vi "SR830Monitor_old.vi"() -> ()   [LabVIEW 2016]
doc: "This VI is an example of storing and recovering data from the SR830 data buffers .\nDATA STORAGE RATE specifes the rate at which data is added to the data buffers .\nSCAN LENGTH specifies the approximate length of the data acquisition scan is seconds .\nPLOT GRAPH, PLOT CH 1 DATA and PLOT CH 2 DATA specify if the respective graphs will be displayed .\nAfter data storage is completed , the channel 1 and channel 2 points are downloaded from the instrument to the CH 1 POINTS and CH 2 POINTS arrays respectively . \nSince data recovered (using the SR830 receive message.vi) is in the string format , this VI requires a considerable amount of time to format the data into an array of floating point numbers . A quicker way would be to store the string in a file and use a CIN to speed up the process ."
uses:
  Global/Global Variables/Data_Display_global.vi
  Instrument_Setup.vi
panel:
  out "AutoSet3":bool=TRUE
  out "AutoSet2":bool=TRUE
  out "AutoSet1":bool=TRUE
  in  "Stopp":bool
  out "error out":T1
  in  "error in":T1
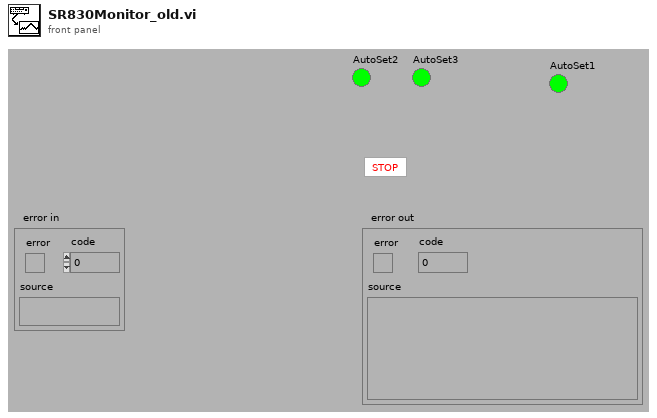
[diagram p1: front panel]
types:
  T1 = cluster{"error":bool, "code":i8, "source":string}
  T2 = cluster{"Lockin1":dbl[], "Lockin3":dbl[], "Lockin2":dbl[]}
  T3 = cluster{"error":bool, "code":i32, "source":string}
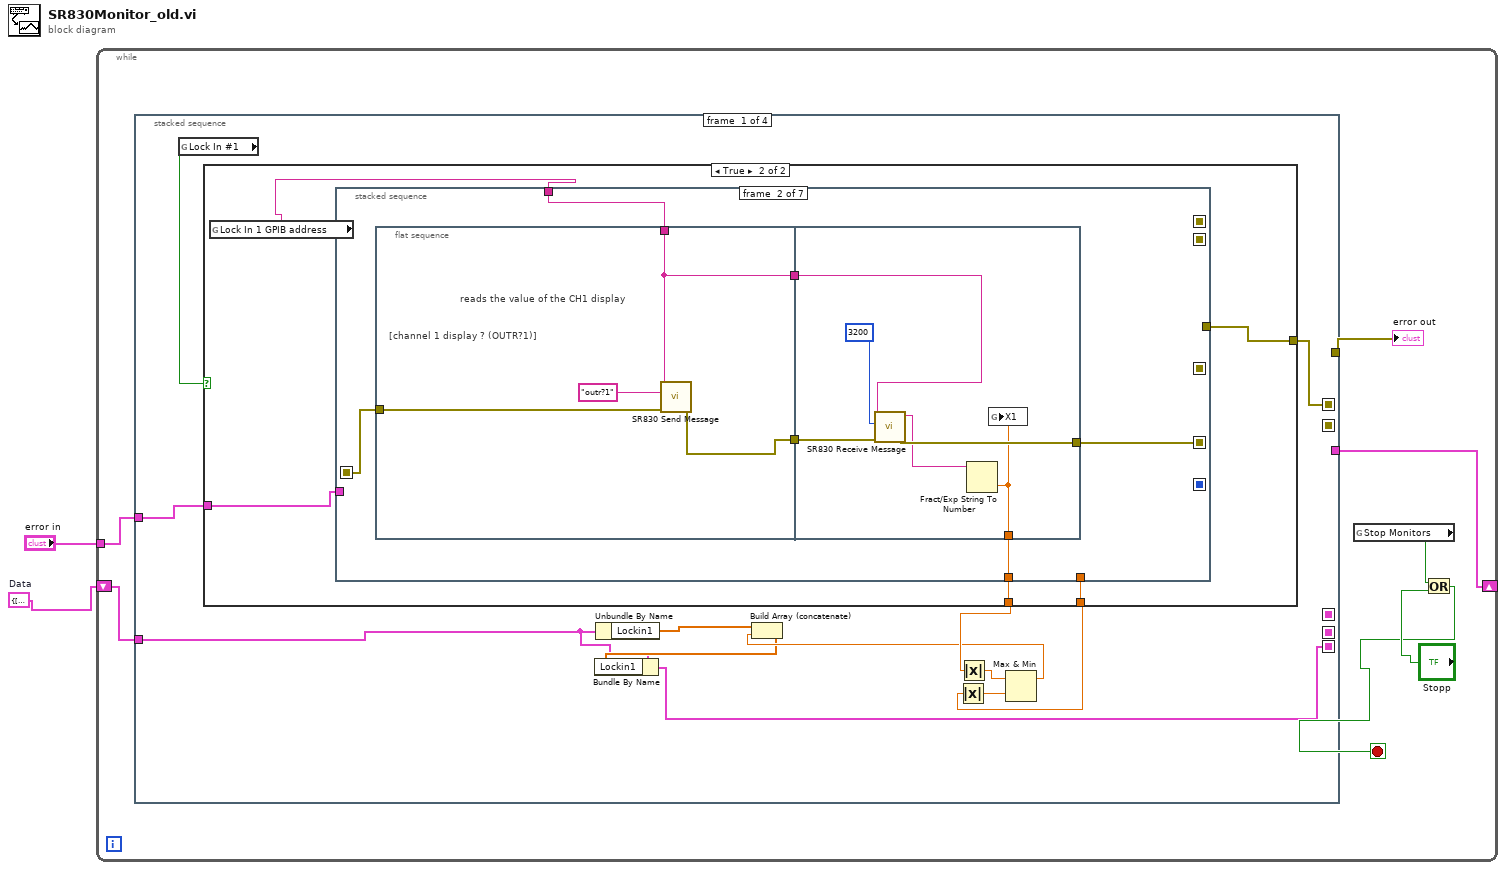
[diagram p0: block diagram]
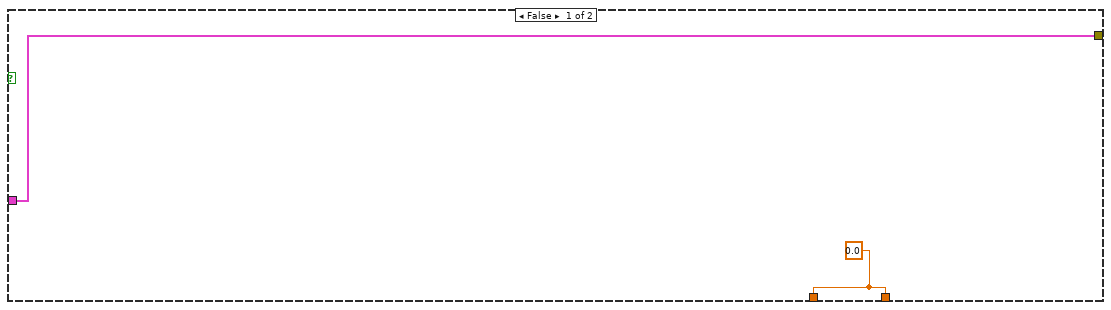
[diagram p2: hidden frame]
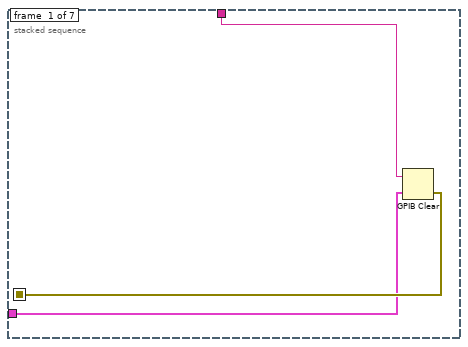
[diagram p3: hidden frame]
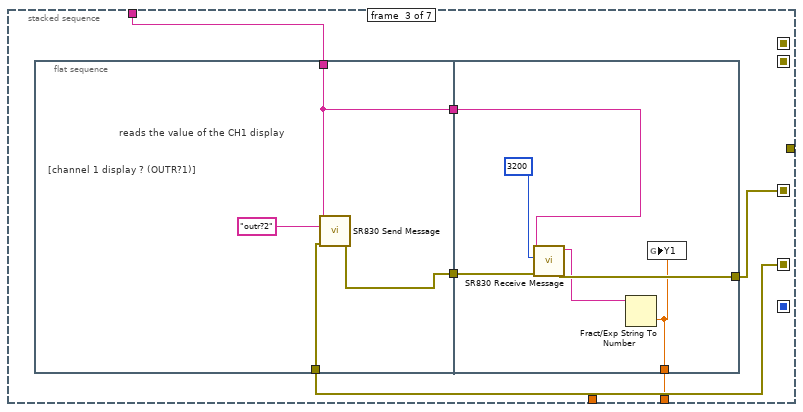
[diagram p4: hidden frame]
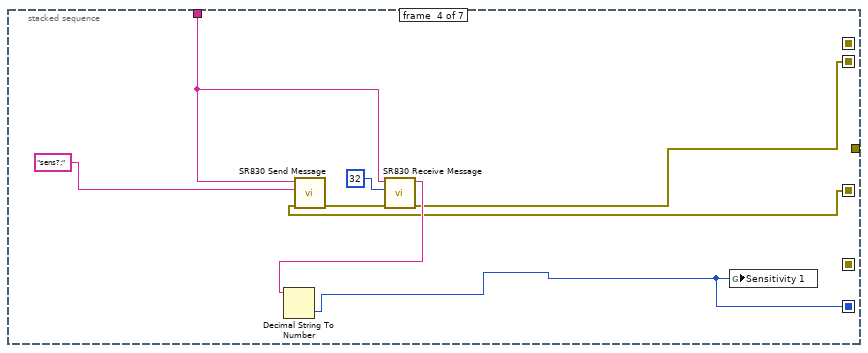
[diagram p5: hidden frame]
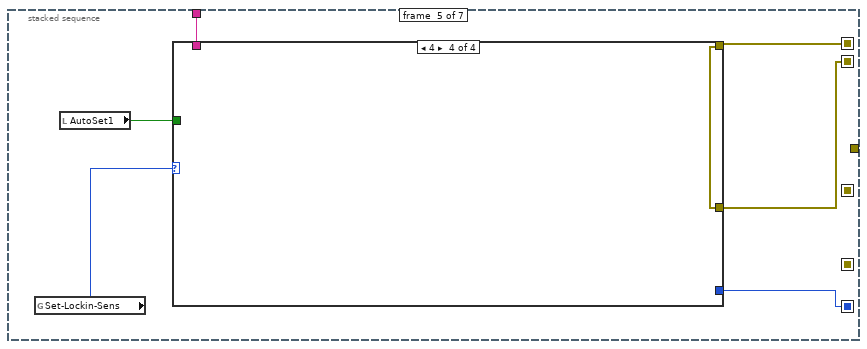
[diagram p6: hidden frame]
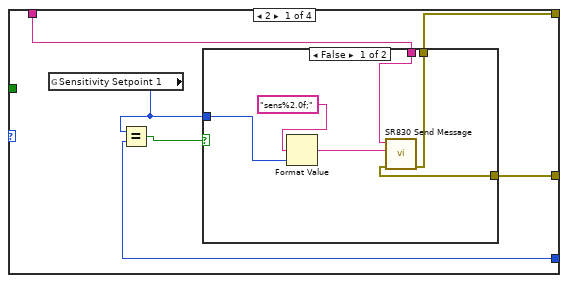
[diagram p7: hidden frame]
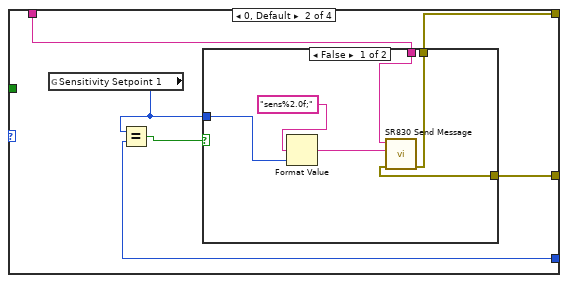
[diagram p9: hidden frame]
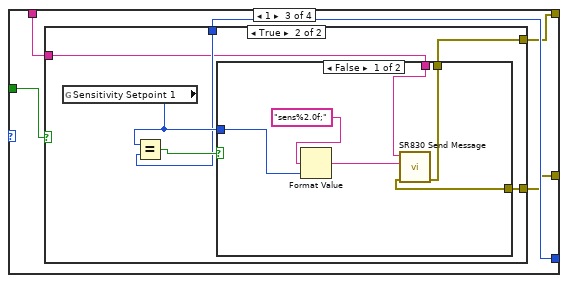
[diagram p11: hidden frame]
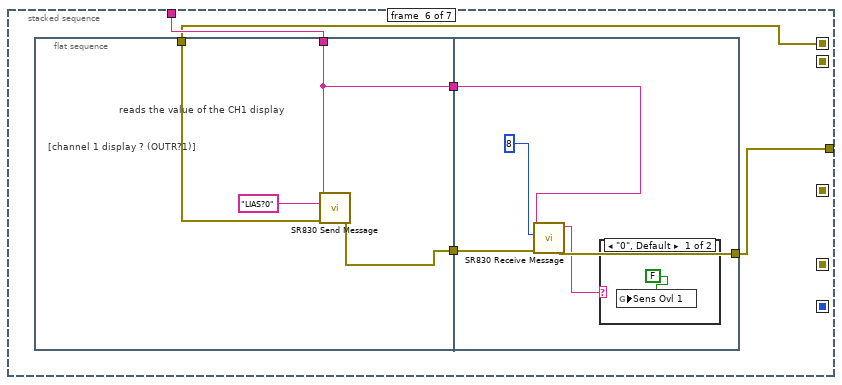
[diagram p14: hidden frame]
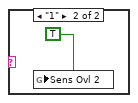
[diagram p15: hidden frame]
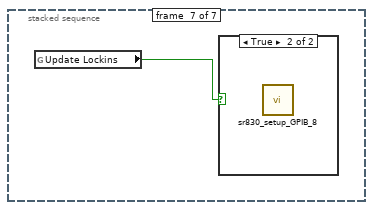
[diagram p16: hidden frame]
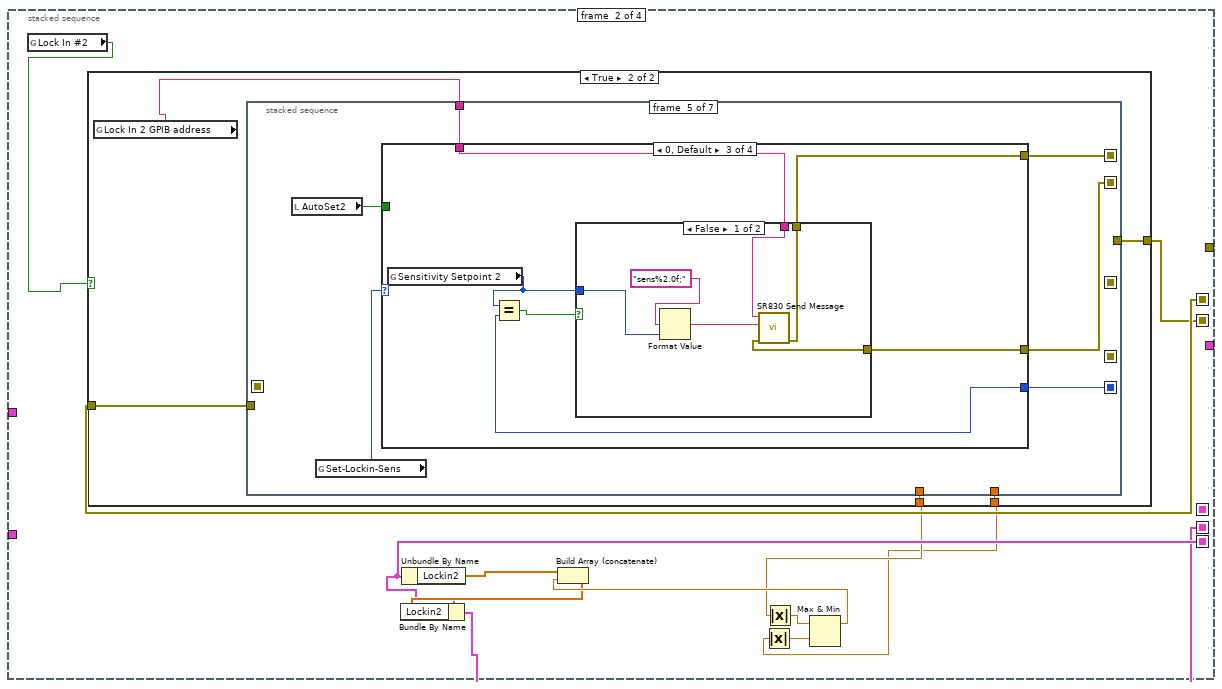
[diagram p18: hidden frame]
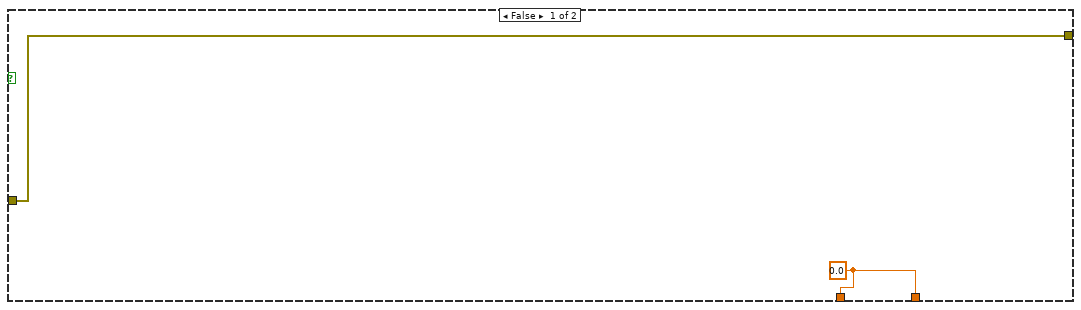
[diagram p19: hidden frame]
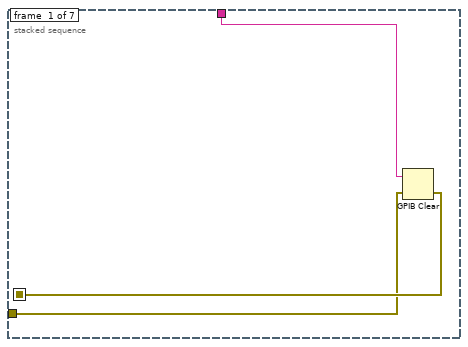
[diagram p20: hidden frame]
diagram:
  w1 = T2 {"Lockin1"=[], "Lockin3"=[], "Lockin2"=[]}  # Data
  n1 = while {
    tunnel: "error in" -> [w9]
    shift-right: [w3] -> _
    shift-left: w1 -> [w4]
    stop <- w5 stop-if-true
    n2 = stacked-sequence {
      seq-local: [w19 _ _ _] -> [_ w152 w284 _]
      seq-local: [_ w150 _ _] -> [_ _ _ _]
      seq-local: [w10 _ _ _] -> [_ w144 _ _]
      seq-local: [_ w141 _ _] -> [_ _ w276 _]
      seq-local: [_ _ w275 _] -> [_ _ _ w391]
      tunnel: w9 -> [w20 _ _ _]
      tunnel: [_ _ w283 _] -> w8
      tunnel: w4 -> [w11 _ _ _]
      tunnel: [_ _ _ w390] -> w3
      frame #0 {
        n3 = global read "Instrument_Setup.vi" "Lock In #1"() -> (w21:bool)
        n4 = case shown="True" w21 {
          tunnel: w20 -> [w23 w28]
          tunnel: [w23 w26] -> w19
          tunnel: [w22 w25] -> w15
          tunnel: [w22 w24] -> w14
          frame False {
            w22 = 0.0
          }
          frame True {
            n5 = global read "Instrument_Setup.vi" "Lock In 1 GPIB address"() -> (w27:string)
            n6 = stacked-sequence {
              seq-local: [_ w34 _ _ _ _ _] -> [_ _ w51 _ _ _ _]
              seq-local: [_ _ w49 _ _ _ _] -> [_ _ _ w66 _ _ _]
              seq-local: [w30 _ _ _ _ _ _] -> [_ w33 _ _ _ _ _]
              seq-local: [_ _ _ w65 _ _ _] -> [_ _ _ _ w77 _ _]
              seq-local: [_ _ _ w64 _ _ _] -> [_ _ _ _ w76 _ _]
              seq-local: [_ _ _ _ w74 _ _] -> [_ _ _ _ _ w124 _]
              tunnel: w27 -> [w31 w37 w50 w68 w75 w126 _]
              tunnel: w28 -> [w29 _ _ _ _ _ _]
              tunnel: [_ _ _ _ _ w125 _] -> w26
              tunnel: [_ w32 _ _ _ _ _] -> w25
              tunnel: [_ _ w48 _ _ _ _] -> w24
              frame #0 {
                n7 = GPIB Clear(2:w29, 3:w31) -> (0:w30:errorcluster)  [unwired: 1 out]
              }
              frame #1 {
                n8 = flat-sequence {
                  tunnel: w37 -> [w40]
                  tunnel: [w40] -> w36
                  tunnel: [w39] -> w35
                  tunnel: w33 -> [w38]
                  tunnel: w36 -> [w46]
                  tunnel: w35 -> [w45]
                  tunnel: [w44] -> w34
                  tunnel: [w42] -> w32
                  frame #0 {
                    # "[channel 1 display ? (OUTR?1)]"
                    # "reads the value of the CH1 display"
                    n9 = call "SR830 Send Message.vi"("address string"=w40, "write buffer"="outr?1", "error in"=w38) -> ("error out"=w39:T3)  [unwired: 4 in, 2 out]
                  }
                  frame #1 {
                    n10 = call "SR830 Receive Message.vi"("address string"=w46, "byte count"=3200, "error in"=w45) -> ("read buffer"=w43:string, "error out"=w44:T3)  [unwired: 4 in, 1 out]
                    n11 = Fract/Exp String To Number(string=w43) -> (number=w42:dbl)  [unwired: 3 in, 1 out]
                    n12 = global write "Data_Display_global.vi" "X1"(w42) -> ()
                  }
                }
              }
              frame #2 {
                n13 = flat-sequence {
                  tunnel: w50 -> [w56]
                  tunnel: [w56] -> w53
                  tunnel: [w55] -> w52
                  tunnel: w51 -> [w54]
                  tunnel: w53 -> [w62]
                  tunnel: w52 -> [w61]
                  tunnel: [w60] -> w49
                  tunnel: [w58] -> w48
                  frame #0 {
                    # "[channel 1 display ? (OUTR?1)]"
                    # "reads the value of the CH1 display"
                    n14 = call "SR830 Send Message.vi"("address string"=w56, "write buffer"="outr?2", "error in"=w54) -> ("error out"=w55:T3)  [unwired: 4 in, 2 out]
                  }
                  frame #1 {
                    n15 = call "SR830 Receive Message.vi"("address string"=w62, "byte count"=3200, "error in"=w61) -> ("read buffer"=w59:string, "error out"=w60:T3)  [unwired: 4 in, 1 out]
                    n16 = Fract/Exp String To Number(string=w59) -> (number=w58:dbl)  [unwired: 3 in, 1 out]
                    n17 = global write "Data_Display_global.vi" "Y1"(w58) -> ()
                  }
                }
              }
              frame #3 {
                n18 = call "SR830 Send Message.vi"("address string"=w68, "write buffer"="sens?;", "error in"=w66) -> ("error out"=w70:T3)  [unwired: 4 in, 2 out]
                n19 = call "SR830 Receive Message.vi"("address string"=w68, "byte count"=32, "error in"=w70) -> ("read buffer"=w67:string, "error out"=w65:T3)  [unwired: 4 in, 1 out]
                n20 = Decimal String To Number(string=w67) -> (number=w64:i32)  [unwired: 2 in, 1 out]
                n21 = global write "Data_Display_global.vi" "Sensitivity 1"(w64) -> ()
              }
              frame #4 {
                n22 = global read "Instrument_Setup.vi" "Set-Lockin-Sens"() -> (w73:u16)
                n23 = local read "AutoSet1"() -> (w72:bool)
                n24 = case shown="4" w73 {
                  tunnel: w77 -> [w81 w94 w104 w123]
                  tunnel: w76 -> [w80 w93 w107 _]
                  tunnel: w75 -> [w79 w92 w106 _]
                  tunnel: [w78 w91 w105 w123] -> w74
                  tunnel: w72 -> [_ _ w108 _]
                  frame 2 {
                    n25 = global read "Data_Display_global.vi" "Sensitivity Setpoint 1"() -> (w82:i32)
                    n26 = Equal?(x=w82, y=w80) -> (x = y?=w83:bool)
                    n27 = case shown="False" w83 {
                      tunnel: w79 -> [w89 _]
                      tunnel: w82 -> [w88 _]
                      tunnel: w81 -> [w87 w90]
                      tunnel: [w86 w90] -> w78
                      frame False {
                        n28 = Format Value(format string="sens%2.0f;", value (0)=w88) -> (output string=w85:string)  [unwired: 1 in]
                        n29 = call "SR830 Send Message.vi"("address string"=w89, "write buffer"=w85, "error in"=w87) -> ("error out"=w86:T3)  [unwired: 4 in, 2 out]
                      }
                      frame True {
                      }
                    }
                  }
                  frame 0, Default {
                    n30 = global read "Data_Display_global.vi" "Sensitivity Setpoint 1"() -> (w95:i32)
                    n31 = Equal?(x=w95, y=w93) -> (x = y?=w96:bool)
                    n32 = case shown="False" w96 {
                      tunnel: w92 -> [w102 _]
                      tunnel: w95 -> [w101 _]
                      tunnel: w94 -> [w100 w103]
                      tunnel: [w99 w103] -> w91
                      frame False {
                        n33 = Format Value(format string="sens%2.0f;", value (0)=w101) -> (output string=w98:string)  [unwired: 1 in]
                        n34 = call "SR830 Send Message.vi"("address string"=w102, "write buffer"=w98, "error in"=w100) -> ("error out"=w99:T3)  [unwired: 4 in, 2 out]
                      }
                      frame True {
                      }
                    }
                  }
                  frame 1 {
                    n35 = case shown="True" w108 {
                      tunnel: w107 -> [_ w113]
                      tunnel: w106 -> [_ w112]
                      tunnel: [w109 w111] -> w105
                      tunnel: w104 -> [w109 w110]
                      frame False {
                      }
                      frame True {
                        n36 = global read "Data_Display_global.vi" "Sensitivity Setpoint 1"() -> (w114:i32)
                        n37 = Equal?(x=w114, y=w113) -> (x = y?=w115:bool)
                        n38 = case shown="False" w115 {
                          tunnel: w112 -> [w121 _]
                          tunnel: w114 -> [w120 _]
                          tunnel: w110 -> [w116 w122]
                          tunnel: [w119 w122] -> w111
                          frame False {
                            n39 = Format Value(format string="sens%2.0f;", value (0)=w120) -> (output string=w118:string)  [unwired: 1 in]
                            n40 = call "SR830 Send Message.vi"("address string"=w121, "write buffer"=w118, "error in"=w116) -> ("error out"=w119:T3)  [unwired: 4 in, 2 out]
                          }
                          frame True {
                          }
                        }
                      }
                    }
                  }
                  frame 4 {
                  }
                }
              }
              frame #5 {
                n41 = flat-sequence {
                  tunnel: w126 -> [w131]
                  tunnel: [w131] -> w128
                  tunnel: [w130] -> w127
                  tunnel: w124 -> [w129]
                  tunnel: w128 -> [w136]
                  tunnel: w127 -> [w135]
                  tunnel: [w134] -> w125
                  frame #0 {
                    # "[channel 1 display ? (OUTR?1)]"
                    # "reads the value of the CH1 display"
                    n42 = call "SR830 Send Message.vi"("address string"=w131, "write buffer"="LIAS?0", "error in"=w129) -> ("error out"=w130:T3)  [unwired: 4 in, 2 out]
                  }
                  frame #1 {
                    n43 = call "SR830 Receive Message.vi"("address string"=w136, "byte count"=8, "error in"=w135) -> ("read buffer"=w133:string, "error out"=w134:T3)  [unwired: 4 in, 1 out]
                    n44 = case shown="\"0\", Default" w133 {
                      frame "0", Default {
                        n45 = global write "Data_Display_global.vi" "Sens Ovl 1"(FALSE) -> ()
                      }
                      frame "1" {
                        n46 = global write "Data_Display_global.vi" "Sens Ovl 2"(TRUE) -> ()
                      }
                    }
                  }
                }
              }
              frame #6 {
                n47 = global read "Instrument_Setup.vi" "Update Lockins"() -> (w140:bool)
                n48 = case shown="True" w140 {
                  frame False {
                  }
                  frame True {
                    n49 = call "sr830_setup_GPIB_8.vi"() -> ()  [unwired: 3 in]
                  }
                }
              }
            }
          }
        }
        n50 = Unbundle By Name(w11) -> ("Lockin1"=w18:dbl[])
        n51 = Absolute Value(x=w14) -> (abs(x)=w16:dbl)
        n52 = Absolute Value(x=w15) -> (abs(x)=w17:dbl)
        n53 = Max & Min(x=w17, y=w16) -> (max(x,y)=w13:dbl)  [unwired: 1 out]
        n54 = Build Array (concatenate)(w18, w13) -> (w12:dbl[])
        n55 = Bundle By Name(cluster=w11, "Lockin1"=w12) -> (w10:T2)
      }
      frame #1 {
        n56 = global read "Instrument_Setup.vi" "Lock In #2"() -> (w151:bool)
        n57 = case shown="True" w151 {
          tunnel: w152 -> [w154 w158]
          tunnel: [w154 w157] -> w150
          tunnel: [w153 w156] -> w143
          tunnel: [w153 w155] -> w142
          frame False {
            w153 = 0.0
          }
          frame True {
            n58 = global read "Instrument_Setup.vi" "Lock In 2 GPIB address"() -> (w159:string)
            n59 = stacked-sequence {
              seq-local: [_ w165 _ _ _ _ _] -> [_ _ w182 _ _ _ _]
              seq-local: [_ _ w180 _ _ _ _] -> [_ _ _ w197 _ _ _]
              seq-local: [w161 _ _ _ _ _ _] -> [_ w164 _ _ _ _ _]
              seq-local: [_ _ _ w196 _ _ _] -> [_ _ _ _ w206 _ _]
              seq-local: [_ _ _ w195 _ _ _] -> [_ _ _ _ w207 _ _]
              seq-local: [_ _ _ _ w205 _ _] -> [_ _ _ _ _ w255 _]
              tunnel: w159 -> [w162 w168 w181 w199 w208 w257 _]
              tunnel: w158 -> [w160 _ _ _ _ _ _]
              tunnel: [_ _ _ _ _ w256 _] -> w157
              tunnel: [_ w163 _ _ _ _ _] -> w156
              tunnel: [_ _ w179 _ _ _ _] -> w155
              frame #0 {
                n60 = GPIB Clear(2:w160, 3:w162) -> (0:w161:errorcluster)  [unwired: 1 out]
              }
              frame #1 {
                n61 = flat-sequence {
                  tunnel: w168 -> [w171]
                  tunnel: [w171] -> w167
                  tunnel: [w170] -> w166
                  tunnel: w164 -> [w169]
                  tunnel: w167 -> [w177]
                  tunnel: w166 -> [w176]
                  tunnel: [w175] -> w165
                  tunnel: [w173] -> w163
                  frame #0 {
                    # "[channel 1 display ? (OUTR?1)]"
                    # "reads the value of the CH1 display"
                    n62 = call "SR830 Send Message.vi"("address string"=w171, "write buffer"="outr?1", "error in"=w169) -> ("error out"=w170:T3)  [unwired: 4 in, 2 out]
                  }
                  frame #1 {
                    n63 = call "SR830 Receive Message.vi"("address string"=w177, "byte count"=3200, "error in"=w176) -> ("read buffer"=w174:string, "error out"=w175:T3)  [unwired: 4 in, 1 out]
                    n64 = Fract/Exp String To Number(string=w174) -> (number=w173:dbl)  [unwired: 3 in, 1 out]
                    n65 = global write "Data_Display_global.vi" "X2"(w173) -> ()
                  }
                }
              }
              frame #2 {
                n66 = flat-sequence {
                  tunnel: w181 -> [w187]
                  tunnel: [w187] -> w184
                  tunnel: [w186] -> w183
                  tunnel: w182 -> [w185]
                  tunnel: w184 -> [w193]
                  tunnel: w183 -> [w192]
                  tunnel: [w191] -> w180
                  tunnel: [w189] -> w179
                  frame #0 {
                    # "[channel 1 display ? (OUTR?1)]"
                    # "reads the value of the CH1 display"
                    n67 = call "SR830 Send Message.vi"("address string"=w187, "write buffer"="outr?2", "error in"=w185) -> ("error out"=w186:T3)  [unwired: 4 in, 2 out]
                  }
                  frame #1 {
                    n68 = call "SR830 Receive Message.vi"("address string"=w193, "byte count"=3200, "error in"=w192) -> ("read buffer"=w190:string, "error out"=w191:T3)  [unwired: 4 in, 1 out]
                    n69 = Fract/Exp String To Number(string=w190) -> (number=w189:dbl)  [unwired: 3 in, 1 out]
                    n70 = global write "Data_Display_global.vi" "Y2"(w189) -> ()
                  }
                }
              }
              frame #3 {
                n71 = call "SR830 Send Message.vi"("address string"=w199, "write buffer"="sens?;", "error in"=w197) -> ("error out"=w201:T3)  [unwired: 4 in, 2 out]
                n72 = call "SR830 Receive Message.vi"("address string"=w199, "byte count"=32, "error in"=w201) -> ("read buffer"=w198:string, "error out"=w196:T3)  [unwired: 4 in, 1 out]
                n73 = Decimal String To Number(string=w198) -> (number=w195:i32)  [unwired: 2 in, 1 out]
                n74 = global write "Data_Display_global.vi" "Sensitivity 2"(w195) -> ()
              }
              frame #4 {
                n75 = local read "AutoSet2"() -> (w203:bool)
                n76 = global read "Instrument_Setup.vi" "Set-Lockin-Sens"() -> (w204:u16)
                n77 = case shown="0, Default" w204 {
                  tunnel: w208 -> [_ w213 w226 w239]
                  tunnel: w207 -> [_ w212 w225 w238]
                  tunnel: w206 -> [w209 w211 w224 w237]
                  tunnel: [w209 w210 w223 w236] -> w205
                  tunnel: w203 -> [_ _ _ w240]
                  frame 4 {
                  }
                  frame 2 {
                    n78 = global read "Data_Display_global.vi" "Sensitivity Setpoint 2"() -> (w214:i32)
                    n79 = Equal?(x=w214, y=w212) -> (x = y?=w215:bool)
                    n80 = case shown="False" w215 {
                      tunnel: w213 -> [w221 _]
                      tunnel: w214 -> [w220 _]
                      tunnel: w211 -> [w219 w222]
                      tunnel: [w218 w222] -> w210
                      frame False {
                        n81 = Format Value(format string="sens%2.0f;", value (0)=w220) -> (output string=w217:string)  [unwired: 1 in]
                        n82 = call "SR830 Send Message.vi"("address string"=w221, "write buffer"=w217, "error in"=w219) -> ("error out"=w218:T3)  [unwired: 4 in, 2 out]
                      }
                      frame True {
                      }
                    }
                  }
                  frame 0, Default {
                    n83 = global read "Data_Display_global.vi" "Sensitivity Setpoint 2"() -> (w227:i32)
                    n84 = Equal?(x=w227, y=w225) -> (x = y?=w228:bool)
                    n85 = case shown="False" w228 {
                      tunnel: w226 -> [w234 _]
                      tunnel: w227 -> [w233 _]
                      tunnel: w224 -> [w232 w235]
                      tunnel: [w231 w235] -> w223
                      frame False {
                        n86 = Format Value(format string="sens%2.0f;", value (0)=w233) -> (output string=w230:string)  [unwired: 1 in]
                        n87 = call "SR830 Send Message.vi"("address string"=w234, "write buffer"=w230, "error in"=w232) -> ("error out"=w231:T3)  [unwired: 4 in, 2 out]
                      }
                      frame True {
                      }
                    }
                  }
                  frame 1 {
                    n88 = case shown="True" w240 {
                      tunnel: w238 -> [_ w245]
                      tunnel: w239 -> [_ w244]
                      tunnel: [w241 w243] -> w236
                      tunnel: w237 -> [w241 w242]
                      frame False {
                      }
                      frame True {
                        n89 = global read "Data_Display_global.vi" "Sensitivity Setpoint 2"() -> (w246:i32)
                        n90 = Equal?(x=w246, y=w245) -> (x = y?=w247:bool)
                        n91 = case shown="True" w247 {
                          tunnel: w244 -> [w253 _]
                          tunnel: w246 -> [w252 _]
                          tunnel: w242 -> [w248 w254]
                          tunnel: [w251 w254] -> w243
                          frame False {
                            n92 = Format Value(format string="sens%2.0f;", value (0)=w252) -> (output string=w250:string)  [unwired: 1 in]
                            n93 = call "SR830 Send Message.vi"("address string"=w253, "write buffer"=w250, "error in"=w248) -> ("error out"=w251:T3)  [unwired: 4 in, 2 out]
                          }
                          frame True {
                          }
                        }
                      }
                    }
                  }
                }
              }
              frame #5 {
                n94 = flat-sequence {
                  tunnel: w257 -> [w262]
                  tunnel: [w262] -> w259
                  tunnel: [w261] -> w258
                  tunnel: w255 -> [w260]
                  tunnel: w259 -> [w267]
                  tunnel: w258 -> [w266]
                  tunnel: [w265] -> w256
                  frame #0 {
                    # "[channel 1 display ? (OUTR?1)]"
                    # "reads the value of the CH1 display"
                    n95 = call "SR830 Send Message.vi"("address string"=w262, "write buffer"="LIAS?0", "error in"=w260) -> ("error out"=w261:T3)  [unwired: 4 in, 2 out]
                  }
                  frame #1 {
                    n96 = call "SR830 Receive Message.vi"("address string"=w267, "byte count"=8, "error in"=w266) -> ("read buffer"=w264:string, "error out"=w265:T3)  [unwired: 4 in, 1 out]
                    n97 = case shown="\"0\", Default" w264 {
                      frame "0", Default {
                        n98 = global write "Data_Display_global.vi" "Sens Ovl 2"(FALSE) -> ()
                      }
                      frame "1" {
                        n99 = global write "Data_Display_global.vi" "Sens Ovl 2"(TRUE) -> ()
                      }
                    }
                  }
                }
              }
              frame #6 {
                n100 = global read "Instrument_Setup.vi" "Update Lockins"() -> (w271:bool)
                n101 = case shown="True" w271 {
                  frame False {
                  }
                  frame True {
                    n102 = flat-sequence {
                      frame #0 {
                        n103 = call "sr830_setup_GPIB_9.vi"() -> ()  [unwired: 3 in]
                      }
                      frame #1 {
                        n104 = global write "Instrument_Setup.vi" "Update Lockins"(FALSE) -> ()
                      }
                    }
                  }
                }
              }
            }
          }
        }
        n105 = Unbundle By Name(w144) -> ("Lockin2"=w149:dbl[])
        n106 = Absolute Value(x=w142) -> (abs(x)=w147:dbl)
        n107 = Absolute Value(x=w143) -> (abs(x)=w148:dbl)
        n108 = Max & Min(x=w148, y=w147) -> (max(x,y)=w146:dbl)  [unwired: 1 out]
        n109 = Build Array (concatenate)(w149, w146) -> (w145:dbl[])
        n110 = Bundle By Name(cluster=w144, "Lockin2"=w145) -> (w141:T2)
      }
      frame #2 {
        n111 = global read "Instrument_Setup.vi" "Lock In #3"() -> (w282:bool)
        n112 = case shown="True" w282 {
          tunnel: w284 -> [w286 w290]
          tunnel: [w286 w291] -> w283
          tunnel: [w285 w288] -> w274
          tunnel: [w285 w287] -> w273
          frame False {
            w285 = 0.0
          }
          frame True {
            n113 = global read "Instrument_Setup.vi" "Lock In 3 GPIB address"() -> (w289:string)
            n114 = stacked-sequence {
              seq-local: [_ w297 _ _ _ _] -> [_ _ w314 _ _ _]
              seq-local: [_ _ w312 _ _ _] -> [_ _ _ w329 _ _]
              seq-local: [w293 _ _ _ _ _] -> [_ w296 _ _ _ _]
              seq-local: [_ _ _ w328 _ _] -> [_ _ _ _ w336 _]
              seq-local: [_ _ _ w327 _ _] -> [_ _ _ _ w337 _]
              seq-local: [_ _ _ _ w335 _] -> [_ _ _ _ _ w374]
              tunnel: w289 -> [w294 w300 w313 w331 w338 w376]
              tunnel: w290 -> [w292 _ _ _ _ _]
              tunnel: [_ _ _ _ _ w375] -> w291
              tunnel: [_ w295 _ _ _ _] -> w288
              tunnel: [_ _ w311 _ _ _] -> w287
              frame #0 {
                n115 = GPIB Clear(2:w292, 3:w294) -> (0:w293:errorcluster)  [unwired: 1 out]
              }
              frame #1 {
                n116 = flat-sequence {
                  tunnel: w300 -> [w303]
                  tunnel: [w303] -> w299
                  tunnel: [w302] -> w298
                  tunnel: w296 -> [w301]
                  tunnel: w299 -> [w309]
                  tunnel: w298 -> [w308]
                  tunnel: [w307] -> w297
                  tunnel: [w305] -> w295
                  frame #0 {
                    # "[channel 1 display ? (OUTR?1)]"
                    # "reads the value of the CH1 display"
                    n117 = call "SR830 Send Message.vi"("address string"=w303, "write buffer"="outr?1", "error in"=w301) -> ("error out"=w302:T3)  [unwired: 4 in, 2 out]
                  }
                  frame #1 {
                    n118 = call "SR830 Receive Message.vi"("address string"=w309, "byte count"=3200, "error in"=w308) -> ("read buffer"=w306:string, "error out"=w307:T3)  [unwired: 4 in, 1 out]
                    n119 = Fract/Exp String To Number(string=w306) -> (number=w305:dbl)  [unwired: 3 in, 1 out]
                    n120 = global write "Data_Display_global.vi" "X3"(w305) -> ()
                  }
                }
              }
              frame #2 {
                n121 = flat-sequence {
                  tunnel: w313 -> [w319]
                  tunnel: [w319] -> w316
                  tunnel: [w318] -> w315
                  tunnel: w314 -> [w317]
                  tunnel: w316 -> [w325]
                  tunnel: w315 -> [w324]
                  tunnel: [w323] -> w312
                  tunnel: [w321] -> w311
                  frame #0 {
                    # "[channel 1 display ? (OUTR?1)]"
                    # "reads the value of the CH1 display"
                    n122 = call "SR830 Send Message.vi"("address string"=w319, "write buffer"="outr?2", "error in"=w317) -> ("error out"=w318:T3)  [unwired: 4 in, 2 out]
                  }
                  frame #1 {
                    n123 = call "SR830 Receive Message.vi"("address string"=w325, "byte count"=3200, "error in"=w324) -> ("read buffer"=w322:string, "error out"=w323:T3)  [unwired: 4 in, 1 out]
                    n124 = Fract/Exp String To Number(string=w322) -> (number=w321:dbl)  [unwired: 3 in, 1 out]
                    n125 = global write "Data_Display_global.vi" "Y3"(w321) -> ()
                  }
                }
              }
              frame #3 {
                n126 = call "SR830 Send Message.vi"("address string"=w331, "write buffer"="sens?;", "error in"=w329) -> ("error out"=w333:T3)  [unwired: 4 in, 2 out]
                n127 = call "SR830 Receive Message.vi"("address string"=w331, "byte count"=32, "error in"=w333) -> ("read buffer"=w330:string, "error out"=w328:T3)  [unwired: 4 in, 1 out]
                n128 = Decimal String To Number(string=w330) -> (number=w327:i32)  [unwired: 2 in, 1 out]
                n129 = global write "Data_Display_global.vi" "Sensitivity 3"(w327) -> ()
              }
              frame #4 {
                n130 = local read "AutoSet3"() -> (w339:bool)
                n131 = global read "Instrument_Setup.vi" "Set-Lockin-Sens"() -> (w340:u16)
                n132 = case shown="2" w340 {
                  tunnel: w338 -> [w344 _ w358]
                  tunnel: w337 -> [w343 _ w357]
                  tunnel: w336 -> [w342 w354 w356]
                  tunnel: [w341 w354 w355] -> w335
                  tunnel: w339 -> [_ _ w359]
                  frame 2 {
                    n133 = global read "Data_Display_global.vi" "Sensitivity Setpoint 2"() -> (w345:i32)
                    n134 = Equal?(x=w345, y=w343) -> (x = y?=w346:bool)
                    n135 = case shown="False" w346 {
                      tunnel: w344 -> [w352 _]
                      tunnel: w345 -> [w351 _]
                      tunnel: w342 -> [w350 w353]
                      tunnel: [w349 w353] -> w341
                      frame False {
                        n136 = Format Value(format string="sens%2.0f;", value (0)=w351) -> (output string=w348:string)  [unwired: 1 in]
                        n137 = call "SR830 Send Message.vi"("address string"=w352, "write buffer"=w348, "error in"=w350) -> ("error out"=w349:T3)  [unwired: 4 in, 2 out]
                      }
                      frame True {
                      }
                    }
                  }
                  frame 0, Default {
                  }
                  frame 1 {
                    n138 = case shown="False" w359 {
                      tunnel: w357 -> [_ w364]
                      tunnel: w358 -> [_ w363]
                      tunnel: [w360 w362] -> w355
                      tunnel: w356 -> [w360 w361]
                      frame False {
                      }
                      frame True {
                        n139 = global read "Data_Display_global.vi" "Sensitivity Setpoint 3"() -> (w365:i32)
                        n140 = Equal?(x=w365, y=w364) -> (x = y?=w366:bool)
                        n141 = case shown="False" w366 {
                          tunnel: w363 -> [w372 _]
                          tunnel: w365 -> [w371 _]
                          tunnel: w361 -> [w367 w373]
                          tunnel: [w370 w373] -> w362
                          frame False {
                            n142 = Format Value(format string="sens%2.0f;", value (0)=w371) -> (output string=w369:string)  [unwired: 1 in]
                            n143 = call "SR830 Send Message.vi"("address string"=w372, "write buffer"=w369, "error in"=w367) -> ("error out"=w370:T3)  [unwired: 4 in, 2 out]
                          }
                          frame True {
                          }
                        }
                      }
                    }
                  }
                }
              }
              frame #5 {
                n144 = flat-sequence {
                  tunnel: w376 -> [w381]
                  tunnel: [w381] -> w378
                  tunnel: [w380] -> w377
                  tunnel: w374 -> [w379]
                  tunnel: w378 -> [w386]
                  tunnel: w377 -> [w385]
                  tunnel: [w384] -> w375
                  frame #0 {
                    # "[channel 1 display ? (OUTR?1)]"
                    # "reads the value of the CH1 display"
                    n145 = call "SR830 Send Message.vi"("address string"=w381, "write buffer"="LIAS?0", "error in"=w379) -> ("error out"=w380:T3)  [unwired: 4 in, 2 out]
                  }
                  frame #1 {
                    n146 = call "SR830 Receive Message.vi"("address string"=w386, "byte count"=8, "error in"=w385) -> ("read buffer"=w383:string, "error out"=w384:T3)  [unwired: 4 in, 1 out]
                    n147 = case shown="\"0\", Default" w383 {
                      frame "0", Default {
                        n148 = global write "Data_Display_global.vi" "Sens Ovl 3"(FALSE) -> ()
                      }
                      frame "1" {
                        n149 = global write "Data_Display_global.vi" "Sens Ovl 2"(TRUE) -> ()
                      }
                    }
                  }
                }
              }
            }
          }
        }
        n150 = Unbundle By Name(w276) -> ("Lockin3"=w281:dbl[])
        n151 = Absolute Value(x=w273) -> (abs(x)=w279:dbl)
        n152 = Absolute Value(x=w274) -> (abs(x)=w280:dbl)
        n153 = Max & Min(x=w280, y=w279) -> (max(x,y)=w278:dbl)  [unwired: 1 out]
        n154 = Build Array (concatenate)(w281, w278) -> (w277:dbl[])
        n155 = Bundle By Name(cluster=w276, "Lockin3"=w277) -> (w275:T2)
      }
      frame #3 {
        n156 = global read "Instrument_Setup.vi" "Set-Lockin-Sens"() -> (w392:u16)
        n157 = case shown="1" w392 {
          tunnel: w391 -> [w396 w416]
          tunnel: w391 -> [_ w413]
          tunnel: [w396 w411] -> w390
          frame 0, Default {
          }
          frame 1 {
            n158 = global read "Data_Display_global.vi" "Sensitivity 1"() -> (w414:i32)
            n159 = Unbundle By Name(w416) -> ("Lockin1"=w415:dbl[], "Lockin2"=w408:dbl[], "Lockin3"=w407:dbl[])
            n160 = global read "Data_Display_global.vi" "Sensitivity 3"() -> (w403:i32)
            n161 = global read "Data_Display_global.vi" "Sensitivity 2"() -> (w404:i32)
            n162 = global read "Instrument_Setup.vi" "Lock In #2"() -> (w398:bool)
            n163 = global read "Instrument_Setup.vi" "Lock In #3"() -> (w397:bool)
            n164 = case shown="False" w398 {
              tunnel: w408 -> [w427 w432]
              tunnel: [w427 w431] -> w406
              tunnel: w404 -> [w426 w430]
              tunnel: [w426 w429] -> w401
              tunnel: [FALSE w428] -> w400
              frame False {
              }
              frame True {
                n165 = call "SR830_AutoSens.vi"("Sensitivity"=w430, "Data in"=w432) -> ("Sensitivity Out"=w429:i32, "Set Sensitivity"=w428:bool, "Data out"=w431:dbl[])  [unwired: 1 in]
              }
            }
            "AutoSet2" <- w400
            n166 = case shown="False" w397 {
              tunnel: w407 -> [w419 w424]
              tunnel: [w419 w423] -> w405
              tunnel: w403 -> [w418 w422]
              tunnel: [w418 w421] -> w402
              tunnel: [FALSE w420] -> w399
              frame False {
              }
              frame True {
                n167 = call "SR830_AutoSens.vi"("Sensitivity"=w422, "Data in"=w424) -> ("Sensitivity Out"=w421:i32, "Set Sensitivity"=w420:bool, "Data out"=w423:dbl[])  [unwired: 1 in]
              }
            }
            "AutoSet3" <- w399
            n168 = call "SR830_AutoSens.vi"("Sensitivity"=w414, "Data in"=w415) -> ("Sensitivity Out"=w409:i32, "Set Sensitivity"=→"AutoSet1":bool, "Data out"=w412:dbl[])  [unwired: 1 in]
            n169 = global write "Data_Display_global.vi" "Sensitivity Setpoint 3"(w402) -> ()
            n170 = global write "Data_Display_global.vi" "Sensitivity Setpoint 2"(w401) -> ()
            n171 = global write "Data_Display_global.vi" "Sensitivity Setpoint 1"(w409) -> ()
            n172 = Bundle By Name(cluster=w413, "Lockin1"=w412, "Lockin2"=w406, "Lockin3"=w405) -> (w411:T2)
          }
        }
        n173 = global read "Instrument_Setup.vi" "Lock-in Readout time"() -> (w395:dbl)
        n174 = Multiply(x=w395, y=1000) -> (x*y=w393:dbl)
        n175 = Wait (ms)(milliseconds to wait=w393) -> ()  [unwired: 1 out]
      }
    }
    "error out" <- w8
    n176 = global read "Data_Display_global.vi" "Stop Monitors"() -> (w7:bool)
    n177 = Or(x=w7, y="Stopp") -> (x .or. y?=w5:bool)
  }
